vi "01_MakeArrayNEW.vi"(0 "Amp":dbl min=0.0, 1 "Step":dbl=0.001 min=0.001, 2 "Bias":dbl, 3 "WaveForm":i32(listbox)) -> (7 "Array":dbl[](array[numeric]), 10 "ArraySize":i32)   [LabVIEW 2017]
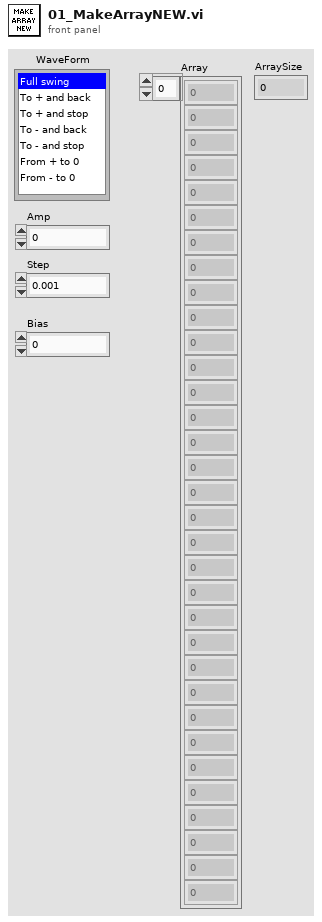
[diagram p1: front panel]
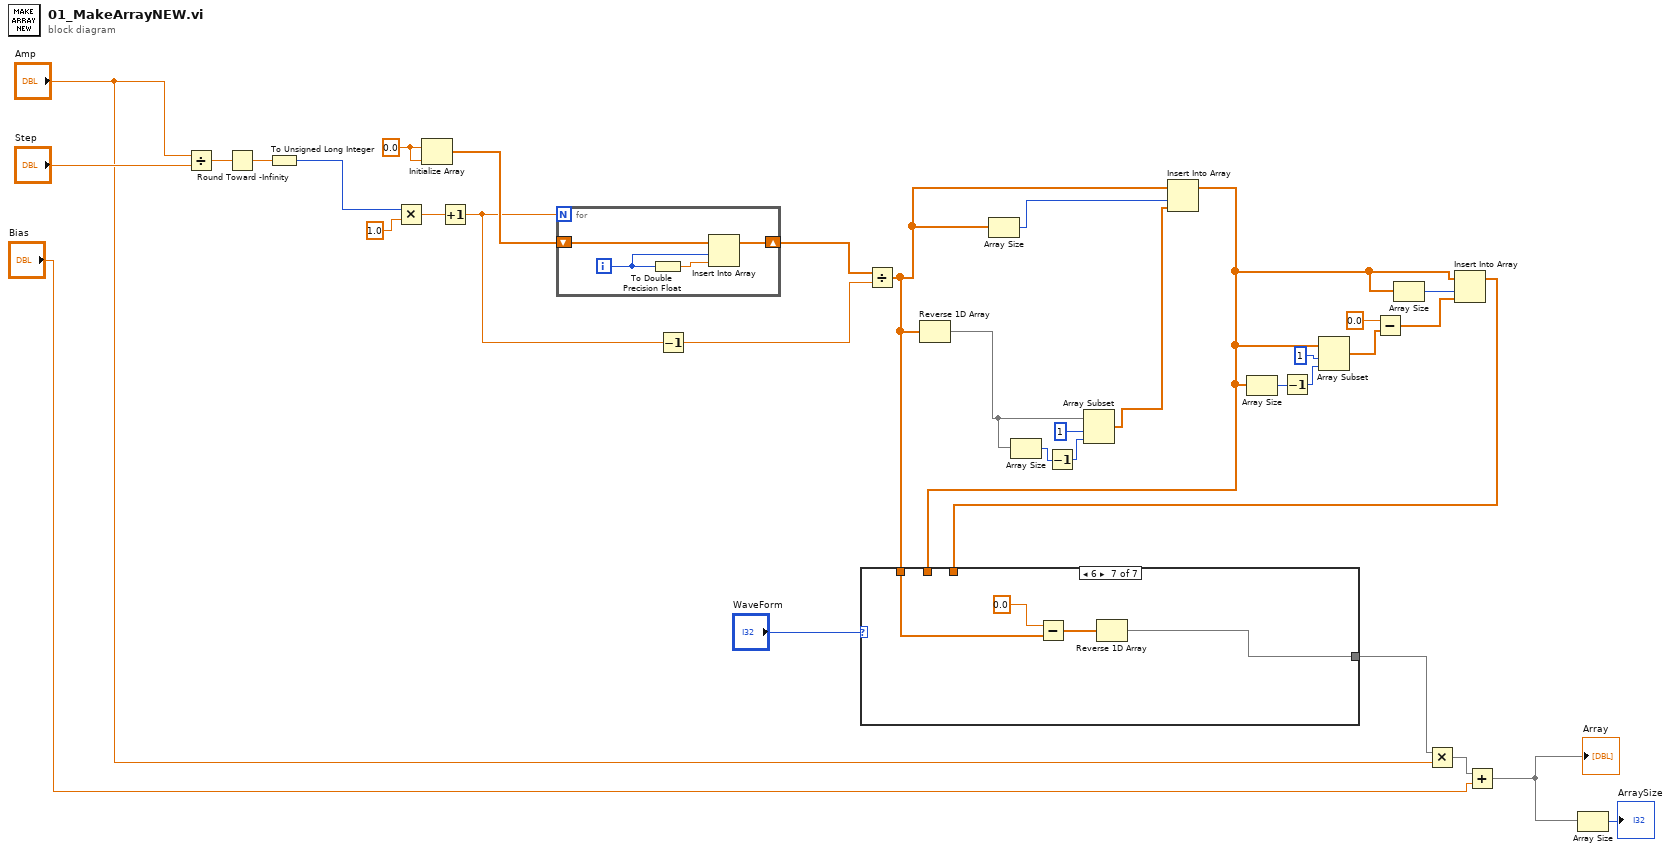
[diagram p0: block diagram]
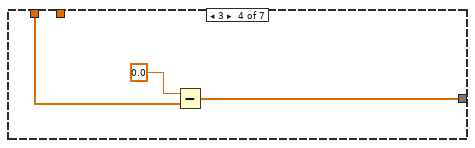
[diagram p5: hidden frame]
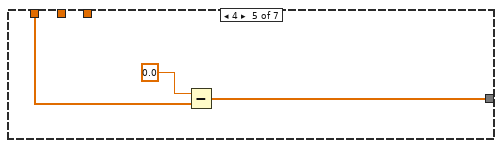
[diagram p6: hidden frame]
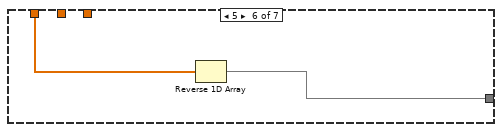
[diagram p7: hidden frame]
diagram:
  w30 = 0.0 ("element")
  n1 = Divide(x="Amp", y="Step") -> (x/y=w33:dbl)
  n2 = Round Toward -Infinity(1:w33) -> (0:w32:dbl)
  n3 = To Unsigned Long Integer(number=w32) -> (unsigned 32bit integer=w28:u32)
  n4 = Multiply(x=w28, y=1.0) -> (x*y=w27:dbl)
  n5 = Initialize Array(w30, w30) -> (w31:dbl[])
  n6 = Increment(x=w27) -> (x+1=w24:dbl)
  n7 = for {
    N: w24 -> [_]
    shift-right: [w37] -> w25
    shift-left: w31 -> [w38]
    i -> [w36]
    n8 = To Double Precision Float(number=w36) -> (double precision float=w35:dbl)
    n9 = Insert Into Array(array=w38, index=w36, new element=w35) -> (w37:dbl[])
  }
  n10 = Decrement(x=w24) -> (x-1=w26:dbl)
  n11 = Divide(x=w25, y=w26) -> (x/y=w9:dbl[])
  n12 = Reverse 1D Array(array=w9) -> (reversed array=w20:dbl[])
  n13 = Array Size(array=w9) -> (size(s)=w18:i32)
  n14 = Array Size(array=w20) -> (size(s)=w21:i32)
  n15 = Decrement(x=w21) -> (x-1=w22:i32)
  n16 = Array Subset(array=w20, index=1, length=w22) -> (w19:dbl[])
  n17 = Insert Into Array(array=w9, index=w18, new element=w19) -> (w8:dbl[])
  n18 = Array Size(array=w8) -> (size(s)=w11:i32)
  n19 = Decrement(x=w11) -> (x-1=w12:i32)
  n20 = Array Subset(array=w8, index=1, length=w12) -> (w14:dbl[])
  n21 = Subtract(x=0.0, y=w14) -> (x-y=w16:dbl[])
  n22 = Array Size(array=w8) -> (size(s)=w15:i32)
  n23 = Insert Into Array(array=w8, index=w15, new element=w16) -> (w7:dbl[])
  n24 = case shown="6" "WaveForm" {
    tunnel: w9 -> [_ _ w41 _ w45 w49 w50]
    tunnel: w8 -> [_ w40 _ w42 _ _ _]
    tunnel: w7 -> [w39 _ _ _ _ _ _]
    tunnel: [w39 w40 w41 w44 w46 w48 w53] -> w6
    frame 0, Default {
    }
    frame 1 {
    }
    frame 2 {
    }
    frame 3 {
      n25 = Subtract(x=0.0, y=w42) -> (x-y=w44:dbl[])
    }
    frame 4 {
      n26 = Subtract(x=0.0, y=w45) -> (x-y=w46:dbl[])
    }
    frame 5 {
      n27 = Reverse 1D Array(array=w49) -> (reversed array=w48:dbl[])
    }
    frame 6 {
      n28 = Subtract(x=0.0, y=w50) -> (x-y=w51:dbl[])
      n29 = Reverse 1D Array(array=w51) -> (reversed array=w53:dbl[])
    }
  }
  n30 = Multiply(x=w6, y="Amp") -> (x*y=w3:dbl[])
  n31 = Add(x=w3, y="Bias") -> (x+y=w2:dbl[])
  "Array" <- w2
  n32 = Array Size(array=w2) -> (size(s)=→"ArraySize":i32)
